vi "Read_from_OPC_UA.vi"() -> ()   [LabVIEW 2021]
uses:
  <vilib>/OPCUA/client/Multiple Read Double.vi
  <vilib>/OPCUA/NI OPC UA Client.lvlib
panel:
  out "Temperature value":dbl
  in  "Node Id":string
  in  "server endpoint URL":string
  in  "stop":bool
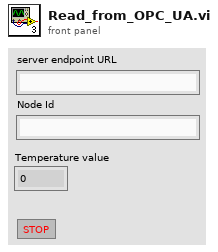
[diagram p1: front panel]
types:
  T1 = cluster{"message mode":enum16{"None", "Sign", "Sign and Encrypt"}, "security":enum16{"Basic256", "Basic128Rsa15"}}
  T2 = typedef "OPC UA Client Refnum.ctl" = refnum<k21>
  T3 = typedef "NodeId.ctl" = string
  T4 = typedef "OPC UA StatusCode.ctl" = u32
  T5 = cluster{"node ID":T3, "value ":dbl, "timestamp":timestamp, "status":T4}[]
  T6 = cluster{"node ID":T3, "value ":dbl, "timestamp":timestamp, "status":T4}
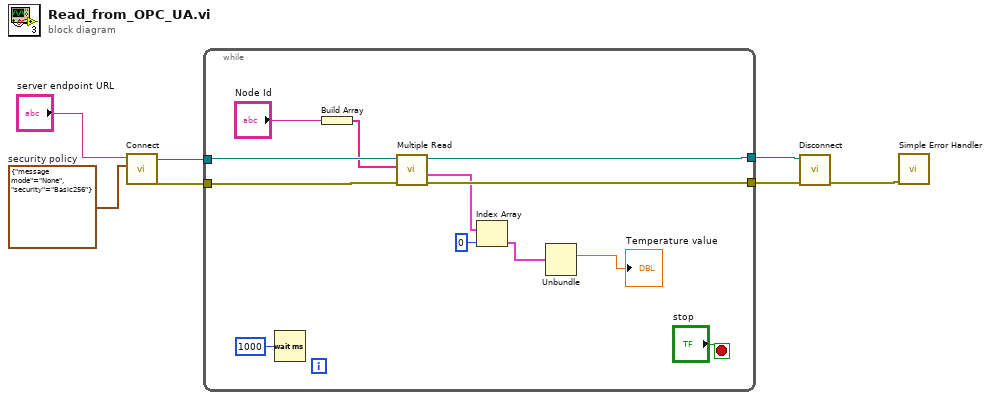
[diagram p0: block diagram]
diagram:
  w7 = T1 {"message mode"=enum."None", "security"=enum."Basic256"}  # security policy
  n1 = call <vilib>:"Connect.vi"("security policy"=w7, "server endpoint URL"="server endpoint URL") -> ("error out"=w4:errorcluster, "OPC UA client refnum out"=w5:T2)  [unwired: 7 in, 1 out]
  n2 = while {
    tunnel: w5 -> [w17]
    tunnel: w4 -> [w15]
    tunnel: [w14] -> w1
    tunnel: [w16] -> w2
    stop <- "stop" stop-if-true
    n3 = Wait (ms)(milliseconds to wait=u32 1000) -> ()  [unwired: 1 out]
    n4 = Build Array("Node Id") -> (w12:string[])
    n5 = call-poly <vilib>:"Multiple Read.vi"("error in (no error)"=w15, "node IDs"=w12, "OPC UA client refnum in"=w17) -> ("error out"=w14:errorcluster, "results"=w10:T5, "OPC UA client refnum out"=w16:T2)  [unwired: 5 in, 1 out]
    n6 = Index Array "Index Array"(array=w10, index=0) -> (element=w9:T6)
    n7 = Unbundle(w9) -> ("value"=→"Temperature value":dbl)  [unwired: 3 out]
  }
  n8 = call <vilib>:"Disconnect.vi"("error in (no error)"=w1, "OPC UA client refnum in"=w2) -> ("error out"=w3:errorcluster)  [unwired: 9 in]
  n9 = call <vilib>:"Simple Error Handler.vi"("error in (no error)"=w3) -> ()  [unwired: 4 in, 5 out]
